vi "SavPath.vi"() -> ()   [LabVIEW 2013]
panel:
  in  "SavePath":path
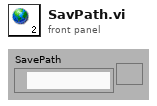
[diagram p1: front panel]
diagram:
